vi "Connect PV.vi"(7 "Commit?":bool, 8 "Error In":errorcluster, 9 "PV TypeDef":string, 10 "PV URL":string, 11 "BNT_SLTagMonitor in":refnum<class "BNT_SLTagMonitor.lvclass">) -> (0 "Error Out":errorcluster, 3 "BNT_SLTagMonitor out":refnum<class "BNT_SLTagMonitor.lvclass">)   [LabVIEW 2019, in "BNT_SLTagMonitor.lvlib" / "BNT_SLTagMonitor.lvclass"]
doc: "Open connection to process variable."
uses:
  BNT_SLTagMonitor.lvclass
  CSPP_Core/Libraries/Utilities/CSPP_Utilities.lvlib
  BNT_SLTools.lvlib
  <vilib>/Skyline/Tag/Wrapper/Wrapper_class/NI Skyline Tag.lvclass
  <vilib>/Skyline/Tag/Wrapper/Wrapper AMQP_class/Query Tags AMQP.vi
  <vilib>/Skyline/Tag/Wrapper/Wrapper AMQP_class/NI Skyline Tag AMQP.lvclass
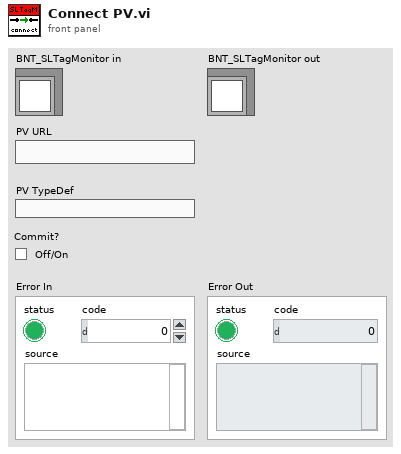
[diagram p1: front panel]
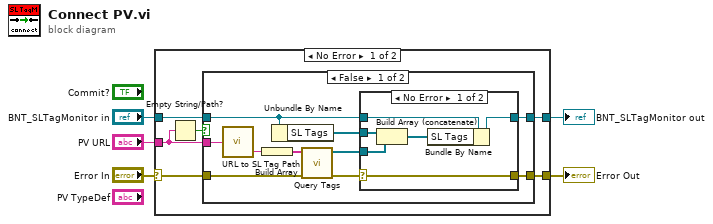
[diagram p0: block diagram]
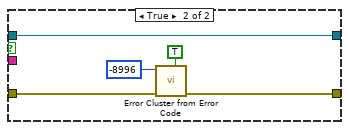
[diagram p3: hidden frame]
diagram:
  n1 = case shown="No Error" "Error In" {
    selector: "Error In" -> [w11 w36]
    tunnel: [w8 w36] -> w2
    tunnel: [w9 w35] -> w4
    tunnel: "BNT_SLTagMonitor in" -> [w10 w35]
    tunnel: "PV URL" -> [w7 _]
    frame No Error {
      n2 = Empty String/Path?(string/path=w7) -> (empty?=w6:bool)
      n3 = case shown="False" w6 {
        tunnel: w11 -> [w16 w32]
        tunnel: w7 -> [w17 _]
        tunnel: w10 -> [w21 w34]
        tunnel: [w20 w34] -> w9
        tunnel: [w18 w31] -> w8
        frame False {
          n4 = call "URL to SL Tag Path.vi"("URL"=w17) -> ("SL Tag Path"=w13:string)
          n5 = Build Array(w13) -> (w12:string[])
          n6 = Unbundle By Name(w21) -> ("SL Tags"=w19:refnum<class "NI Skyline Tag.lvclass">[])
          n7 = call-poly <vilib>:"Query Tags.vi"("error in (no error)"=w16, "paths"=w12) -> ("error out"=w15:errorcluster, "tags"=w14:refnum<class "NI Skyline Tag.lvclass">[])  [unwired: 7 in, 1 out]
          n8 = case shown="No Error" w15 {
            selector: w15 -> [w22 w28]
            tunnel: w14 -> [w27 _]
            tunnel: w21 -> [w26 w29]
            tunnel: [w25 w29] -> w20
            tunnel: w19 -> [w23 _]
            tunnel: [w22 w28] -> w18
            frame No Error {
              n9 = Build Array (concatenate)(w23, w27) -> (w24:refnum<class "NI Skyline Tag.lvclass">[])
              n10 = Bundle By Name(cluster=w26, "SL Tags"=w24) -> (w25:refnum<class "BNT_SLTagMonitor.lvclass">)
            }
            frame Error {
            }
          }
        }
        frame True {
          n11 = call "Error Cluster from Error Code.vi"("is warning? (False)"=TRUE, "Error In"=w32, "Error Code (0)"=-8996 ("error code (no error:0)")) -> ("Error Out"=w31:errorcluster)  [unwired: 8 in]
        }
      }
    }
    frame Error {
    }
  }
  "BNT_SLTagMonitor out" <- w4
  "Error Out" <- w2
